vi "Assert Not Equal Value and Type_Variant.vi"(4 "Execution time (s)":dbl=-1.0, 5 "Assert Only? (F)":bool, 6 "error code (1)":i32=1, 7 "Label":string, 8 "error in (no error)":errorcluster, 10 "Y":variant, 11 "X":variant) -> (0 "error out":errorcluster)   [LabVIEW 2013, in "Caraya.lvlib" / "Assert.lvclass"]
doc: "Generates an error if the input condition is not met.\n\nThis method compares the inputs.\nAsserts TRUE if either type or value of inputs differ.\nAsserts FALSE otherwise.\n\nex 1: Comparing two input integers of equal value and type will assert FALSE.\n\nex 2: Comparing two integer inputs of equal value but of different type representation (U8 and I32) will assert TRUE."
uses:
  Assert.lvclass
  <vilib>/Utility/VariantDataType/VariantType.lvlib
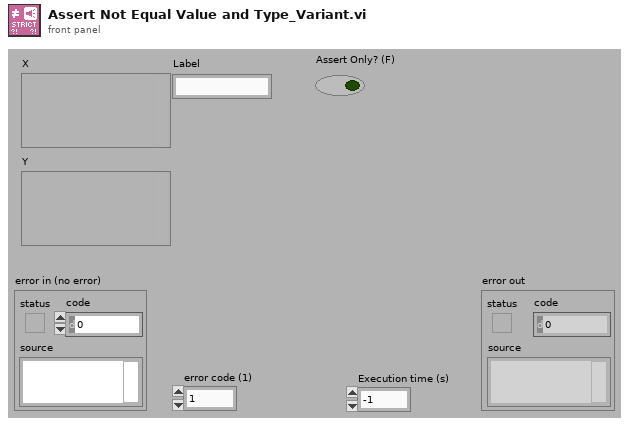
[diagram p1: front panel]
types:
  T1 = typedef "VariantType.lvlib/Type.ctl" = enum8{"Invalid Type", "Void", "I8", "I16", "I32", "I64", "U8", "U16", "U32", "U64", "Single Float", "Double Float", "Extended Float", "Single Complex", "Double Complex", "Extended Complex", "Enum U8", "Enum U16", "Enum U32", "Enum U64", "Single Float With Unit", "Double Float With Unit", "Extended Float With Unit", "Single Complex with Unit", "Double Complex with Unit", "Extended Complex with Unit", "Boolean", "String", "Path", "Picture", "Tag", "Array", "Cluster", "Variant", "LV Variant", "Waveform", "Timestamp", "Digital Waveform", "Digital Data", "ExpressData", "Refnum", "External Data", "VI", "Poly VI", "LabVIEW Class Instance", "Fixed Point"}
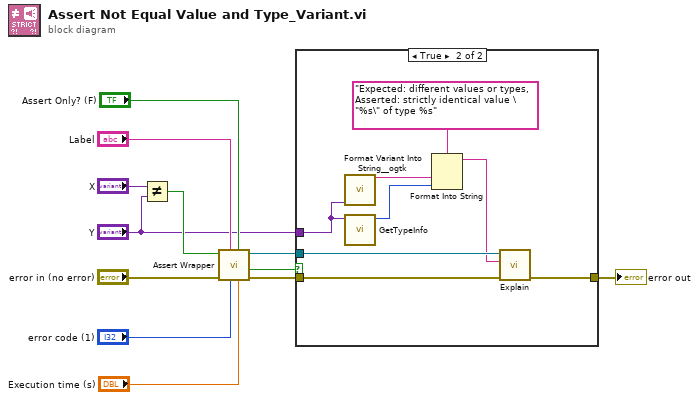
[diagram p0: block diagram]
diagram:
  n1 = Not Equal?(x="X", y="Y") -> (x != y?=w10:bool)
  n2 = call "Assert Wrapper.vi"("Execution time (s)"="Execution time (s)", "Assert Only? (F)"="Assert Only? (F)", "error code (1)"="error code (1)", "Label"="Label", "error in (no error)"="error in (no error)", "Assert?"=w10) -> ("error out"=w6:errorcluster, "Verbose"=w2:bool, "Assert out"=w1:refnum<class "Assert.lvclass">)  [unwired: 3 in]
  n3 = case shown="True" w2 {
    tunnel: [w13 w21] -> w7
    tunnel: w1 -> [_ w20]
    tunnel: w6 -> [w13 w19]
    tunnel: "Y" -> [_ w14]
    frame False {
    }
    frame True {
      n4 = call <userlib>:"Format Variant Into String__ogtk.vi"("Variant"=w14) -> ("Output String"=w17:string)  [unwired: 13 in, 1 out]
      n5 = call <vilib>:"GetTypeInfo.vi"("Variant"=w14) -> ("Type Enum"=w15:T1)  [unwired: 6 in, 4 out]
      n6 = Format Into String(format string="Expected: different values or types, Asserted: strictly identical value \"%s\" of type %s" ("t"), w17, w15) -> (resulting string=w18:string)  [unwired: 2 in, 1 out]
      n7 = call-dynamic "Explain.vi"("error in (no error)"=w19, "Verbose Explanation"=w18, "Assert in"=w20) -> ("error out"=w21:errorcluster)  [unwired: 7 in, 1 out]
    }
  }
  "error out" <- w7
